vi "LV to ITX  Retrieve-HY.vi"(0 "File or Folder Path":path=path "P:/expt/PPMS 2 Data/SA03074H-20190112/08-IV curves-SG 2&3@0T", 5 "offset":i32, 7 "length":i32=91, 9 "index":T1={"A"=17, "B"=4, "C"=4, "D"=1, "E"=17, "N1"=3, "N2"=2, "N3"=0, "N4"=0}, 11 "stop":bool, 12 "file contains 2D data?":bool) -> (4 "A vs B":cluster{dbl[], dbl[]}[](graph), 6 "C vs D":cluster{dbl[], dbl[]}[](graph), 8 "E":dbl[][](graph), 10 "N":cluster{"N1":dbl, "N2":dbl, "N3":dbl, "N4":dbl}={"N1"=0.0, "N2"=0.0, "N3"=3631102351.878283, "N4"=3631102351.878283} {"N4" format="%#_6p"; "N3" format="%#_6p"; "N2" format="%#_6p"; "N1" format="%#_6p"}, 14 "Comments":string="IGOR\nX// Date: 1/23/2019 10:40 AM\nX// T sweep, B sweep, BG=11.5V\nX// \nX// T sweep: 4.5K, 5K, 5.5K\nX// B sweep: 7 to 0T, 0.2T step, 0.5T/min\nX// SG 3: 0 ac + dc: 365mV\nX// SG 2: 0 ac + dc: V(B)+(-450mV to 450mV), 0.5mV step, Ramp \nX// V(B)=V(0T)-17mV*|B|, V(0T)=300mV\nX// \nX// S-5:  2mV ac + 0 dc, 11Hz, Sinewave\nX// D-27\nX// V1+/-: 5/28\nX// \nX// prefilter: 60Hz prefilter-off\nX// TC: 500ms, order-2\nX// filter fC (Hz): 0.31831\nX// Vbg: 1\nX// \n\nX// Temp=5.500000\n\nX// \n\nX// B_Field=2.000000\n\nX// \n\nX// B_Field_Rate=0.500000\n\nX// \n\n\n\n\n\n\n\n\n\n\n\n\n\n\n\n\n\n\n\n\n\n\n\n\n\n\n\n\n\n\n\n\n\n\n\n\n\n\n\n\n\n\n\n\nX \nX Display/R 'time.SA03074H.000097'\nX AppendToGraph 'T.SA03074H.000097'\nX AppendToGraph 'B.SA03074H.000097'\nX AppendToGraph 'B_rate.SA03074H.000097'\nX AppendToGraph 'Vsg.SA03074H.000097'\nX AppendToGraph 'X0.SA03074H.000097'\nX AppendToGraph 'Y0.SA03074H.000097'\nX AppendToGraph 'X1.SA03074H.000097'\nX AppendToGraph 'Y1.SA03074H.000097'\nX AppendToGraph 'X2.SA03074H.000097'\nX AppendToGraph 'Y2.SA03074H.000097'\nX AppendToGraph 'X3.SA03074H.000097'\nX AppendToGraph 'Y3.SA03074H.000097'\nX AppendToGraph 'X4.SA03074H.000097'\nX AppendToGraph 'Y4.SA03074H.000097'\nX AppendToGraph 'X5.SA03074H.000097'\nX AppendToGraph 'Y5.SA03074H.000097'\nX AppendToGraph 'X6.SA03074H.000097'\nX AppendToGraph 'Y6.SA03074H.000097'\nX AppendToGraph 'X7.SA03074H.000097'\nX AppendToGraph 'Y7.SA03074H.000097'\nX Label bottom \"x label\"\nX Label left \"y label\"\nX ModifyGraph rgb('time.SA03074H.000097')=(65280,0,0)\nX ModifyGraph rgb('T.SA03074H.000097')=(65280,16896,0)\nX ModifyGraph rgb('B.SA03074H.000097')=(65280,33792,0)\nX ModifyGraph rgb('B_rate.SA03074H.000097')=(65280,50688,0)\nX ModifyGraph rgb('Vsg.SA03074H.000097')=(63488,65280,0)\nX ModifyGraph rgb('X0.SA03074H.000097')=(46592,65280,0)\nX ModifyGraph rgb('Y0.SA03074H.000097')=(29696,65280,0)\nX ModifyGraph rgb('X1.SA03074H.000097')=(12800,65280,0)\nX ModifyGraph rgb('Y1.SA03074H.000097')=(0,65280,4096)\nX ModifyGraph rgb('X2.SA03074H.000097')=(0,65280,20992)\nX ModifyGraph rgb('Y2.SA03074H.000097')=(0,65280,37888)\nX ModifyGraph rgb('X3.SA03074H.000097')=(0,65280,53248)\nX ModifyGraph rgb('Y3.SA03074H.000097')=(0,60928,65280)\nX ModifyGraph rgb('X4.SA03074H.000097')=(0,44032,65280)\nX ModifyGraph rgb('Y4.SA03074H.000097')=(0,27136,65280)\nX ModifyGraph rgb('X5.SA03074H.000097')=(0,10240,65280)\nX ModifyGraph rgb('Y5.SA03074H.000097')=(6656,0,65280)\nX ModifyGraph rgb('X6.SA03074H.000097')=(23552,0,65280)\nX ModifyGraph rgb('Y6.SA03074H.000097')=(40448,0,65280)\nX ModifyGraph rgb('X7.SA03074H.000097')=(57344,0,65280)\nX ModifyGraph rgb('Y7.SA03074H.000097')=(65280,0,56832)\nX Legend/C/N=text0/J \"\\\\s('time.SA03074H.000097') time\\r\\\\s('T.SA03074H.000097') T\\r\\\\s('B.SA03074H.000097') B\\r\\\\s('B_rate.SA03074H.000097') B_rate\\r\\\\s('Vsg.SA03074H.000097') Vsg\\r\\\\s('X0.SA03074H.000097') X0\\r\\\\s('Y0.SA03074H.000097') Y0\\r\\\\s('X1.SA03074H.000097') X1\\r\\\\s('Y1.SA03074H.000097') Y1\\r\\\\s('X2.SA03074H.000097') X2\\r\\\\s('Y2.SA03074H.000097') Y2\\r\\\\s('X3.SA03074H.000097') X3\\r\\\\s('Y3.SA03074H.000097') Y3\\r\\\\s('X4.SA03074H.000097') X4\\r\\\\s('Y4.SA03074H.000097') Y4\\r\\\\s('X5.SA03074H.000097') X5\\r\\\\s('Y5.SA03074H.000097') Y5\\r\\\\s('X6.SA03074H.000097') X6\\r\\\\s('Y6.SA03074H.000097') Y6\\r\\\\s('X7.SA03074H.000097') X7\\r\\\\s('Y7.SA03074H.000097') Y7\"\nX ModifyGraph mirror(bottom)=1\nX ModifyGraph width=216\nX ModifyGraph height={Aspect,0.6}\nX ModifyGraph Log(bottom)=0\nX ModifyGraph Log(left)=0\nX \n")   [LabVIEW 2016]
uses:
  <vilib>/Utility/miscctls.llb/LVOffsetAndMultiplierTypeDef.ctl
  <userlib>/LevyLab/LV to ITX/LVtoITX.lvclass
  <vilib>/Analysis/NI_AALPro.lvlib
panel:
  in  "Offset value":dbl
  in  "Add offset?":bool
  out "size(s)":i32[](array[numeric])=[21, 1801]
  in  "Specify data section ?":bool
  in  "Data length":i32=5000
  in  "Data offset":i32
  in  "Tab Control 2":enum32{"Amplifier settings", "Page 2"}(tab)
  in  "Sensitivity":dbl
  in  "Current gain":dbl
  out "Actual Current Multiplier (A)":dbl=nan
  in  "Voltage gain":dbl
  in  "Exciting voltage":dbl
  out "Actual Conductance Multiplier (S)":dbl=nan
  out "Actual Conductance Multiplier (e2/h)":dbl=nan
  in  "Unit of conductance":u16(ring) items=["Unit: e2/h", "Unit: S", "Multiplier: 1", "Multiplier: Manual input"]
  in  "Manual input":dbl
  in  "Tab Control":enum32{"Curve-Vertical", "Curve-Horizontal"}(tab)=enum."Curve-Horizontal"
  out "Drag V":cluster{dbl[], dbl[]}(graph)={[7.0, 6.8, 6.6, 6.4, 6.2, 6.0, 5.8, 5.6, 5.4, 5.2, 5.0, 4.8, 4.6, 4.4, 4.199999999999999, 4.0, 3.8, 3.5999999999999996, 3.4, 3.1999999999999997, 3.0, 2.8, 2.5999999999999996, 2.3999999999999995, 2.1999999999999993, 2.0], [nan, nan, nan, nan, nan, nan, nan, nan, nan, nan, nan, nan, nan, nan, nan, nan, nan, nan, nan, nan, nan, nan, nan, nan, nan, nan]}
  out "Numeric X":i32=1
  in  "Average width X":i32=1
  out "From X":dbl=-0.2832407407407408 format="%#_4p"
  out "To X":dbl=-0.2827407407407408 format="%#_4p"
  out "Drag V 2":cluster{dbl[], dbl[]}(graph)={[-0.45, -0.4495, -0.449, -0.4485, -0.448, -0.4475, -0.447, -0.4465, -0.446, -0.4455, -0.445, -0.4445, -0.444, -0.4435, -0.443, -0.4425, -0.442, -0.4415, -0.441, -0.4405, -0.44, -0.4395, -0.439, -0.4385, -0.438, -0.4375], [nan, nan, nan, nan, nan, nan, nan, nan, nan, nan, nan, nan, nan, nan, nan, nan, nan, nan, nan, nan, nan, nan, nan, nan, nan, nan]}
  out "Numeric Y":i32=21
  out "To Y":dbl=-0.3885714285714288 format="%#_4p"
  out "From  Y":dbl=3.8114285714285714 format="%#_4p"
  in  "Average width Y":i32=21
  out "Y Scale Multiplier":dbl=1.0
  out "Z Scale Multiplier":dbl=1.0
  in  "D  is time?":bool
  in  "B is time?":bool
  out "time":string[][](table)=[["1/23/2019", "6:37 AM"], ["1/23/2019", "6:47 AM"], ["1/23/2019", "6:57 AM"], ["1/23/2019", "7:07 AM"], ["1/23/2019", "7:16 AM"], ["1/23/2019", "7:26 AM"], ["1/23/2019", "7:36 AM"], ["1/23/2019", "7:45 AM"], ["1/23/2019", "7:55 AM"], ["1/23/2019", "8:05 AM"], ["1/23/2019", "8:15 AM"], ["1/23/2019", "8:24 AM"], ["1/23/2019", "8:34 AM"], ["1/23/2019", "8:44 AM"], ["1/23/2019", "8:54 AM"], ["1/23/2019", "9:03 AM"], ["1/23/2019", "9:13 AM"], ["1/23/2019", "9:23 AM"], ["1/23/2019", "9:32 AM"], ["1/23/2019", "9:42 AM"], ["1/23/2019", "9:52 AM"], ["1/23/2019", "10:02 AM"], ["1/23/2019", "10:11 AM"], ["1/23/2019", "10:21 AM"], ["1/23/2019", "10:31 AM"], ["1/23/2019", "10:40 AM"]]
  in  "Use Folder Index File?":bool
  in  "Generate Folder Index File?":bool
  in  "Ez name":string="I (A)"
  in  "Ey name":string="B (T)"
  in  "Ex name":string="(DC of SG-L)-V(B) (V)"
  in  "C y name":string="C y name"
  in  "D x name":string="D x name"
  in  "A y name":string="I (A)"
  in  "B x name":string="(DC of SG-L)-V(B) (V)"
  out "Index, Wavenames":string[][](table)=[["0", "'time.SA03074H.000097'\n"], ["1", "'T.SA03074H.000097'\n"], ["2", "'B.SA03074H.000097'\n"], ["3", "'B_rate.SA03074H.000097'\n"], ["4", "'Vsg.SA03074H.000097'\n"], ["5", "'X0.SA03074H.000097'\n"], ["6", "'Y0.SA03074H.000097'\n"], ["7", "'X1.SA03074H.000097'\n"], ["8", "'Y1.SA03074H.000097'\n"], ["9", "'X2.SA03074H.000097'\n"], ["10", "'Y2.SA03074H.000097'\n"], ["11", "'X3.SA03074H.000097'\n"], ["12", "'Y3.SA03074H.000097'\n"], ["13", "'X4.SA03074H.000097'\n"], ["14", "'Y4.SA03074H.000097'\n"], ["15", "'X5.SA03074H.000097'\n"], ["16", "'Y5.SA03074H.000097'\n"], ["17", "'X6.SA03074H.000097'\n"], ["18", "'Y6.SA03074H.000097'\n"], ["19", "'X7.SA03074H.000097'\n"], ["20", "'Y7.SA03074H.000097'\n"], ["", ""]]
  in  "recolor traces?":bool
  in  "Ex":T2={"Offset"=-0.45, "Multiplier"=0.0005}
  in  "Ey":T2={"Offset"=7.0, "Multiplier"=-0.2}
  out "Path":path=path "P:/expt/PPMS 2 Data/SA03074H-20190112/11A-SG-L sweep at B 4K~6K/SA03074H.000097.itx"
  out "counter":i32=25
  in  "pattern":string="*.itx"
  # "Add offset to curves?"
  # "Specify data section"
  # "Setting for Conductance caculation"
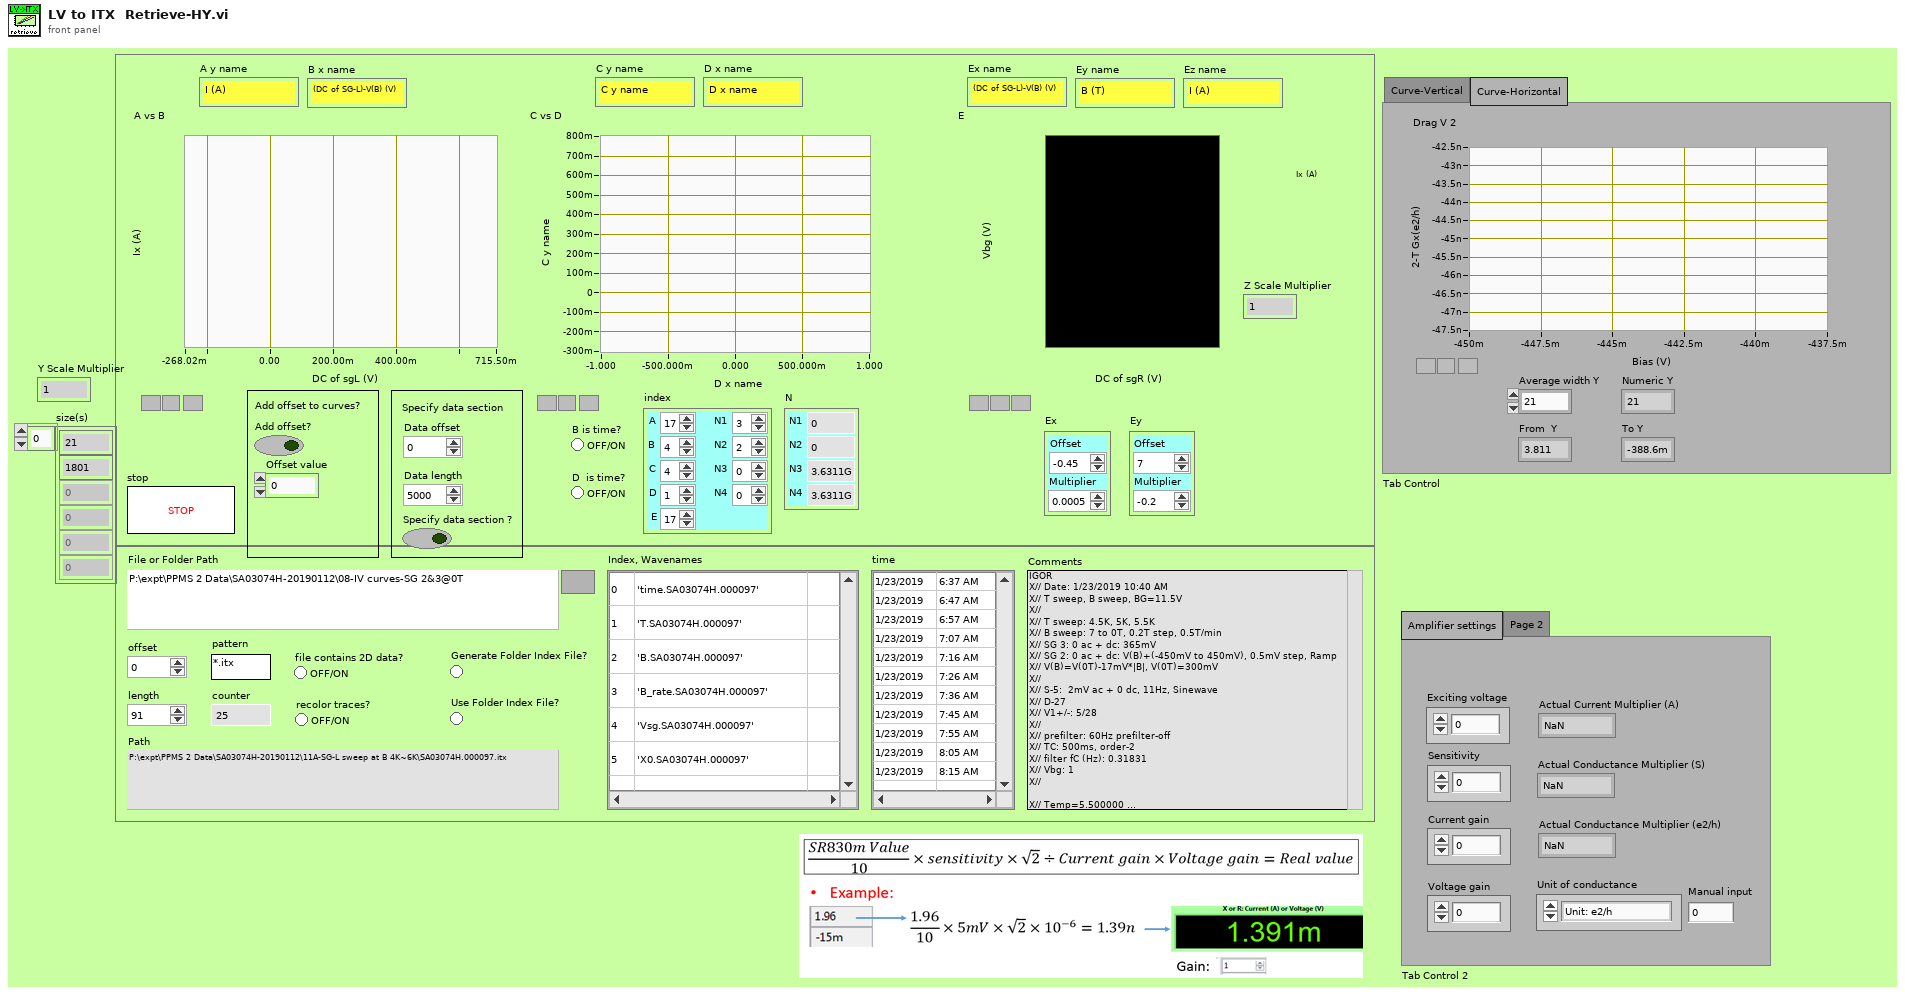
[diagram p1: front panel]
types:
  T1 = cluster{"A":i32, "B":i32, "C":i32, "D":i32, "E":i32, "N1":i32, "N2":i32, "N3":i32, "N4":i32}
  T2 = typedef "LVOffsetAndMultiplierTypeDef.ctl" = cluster{"Offset":dbl, "Multiplier":dbl}
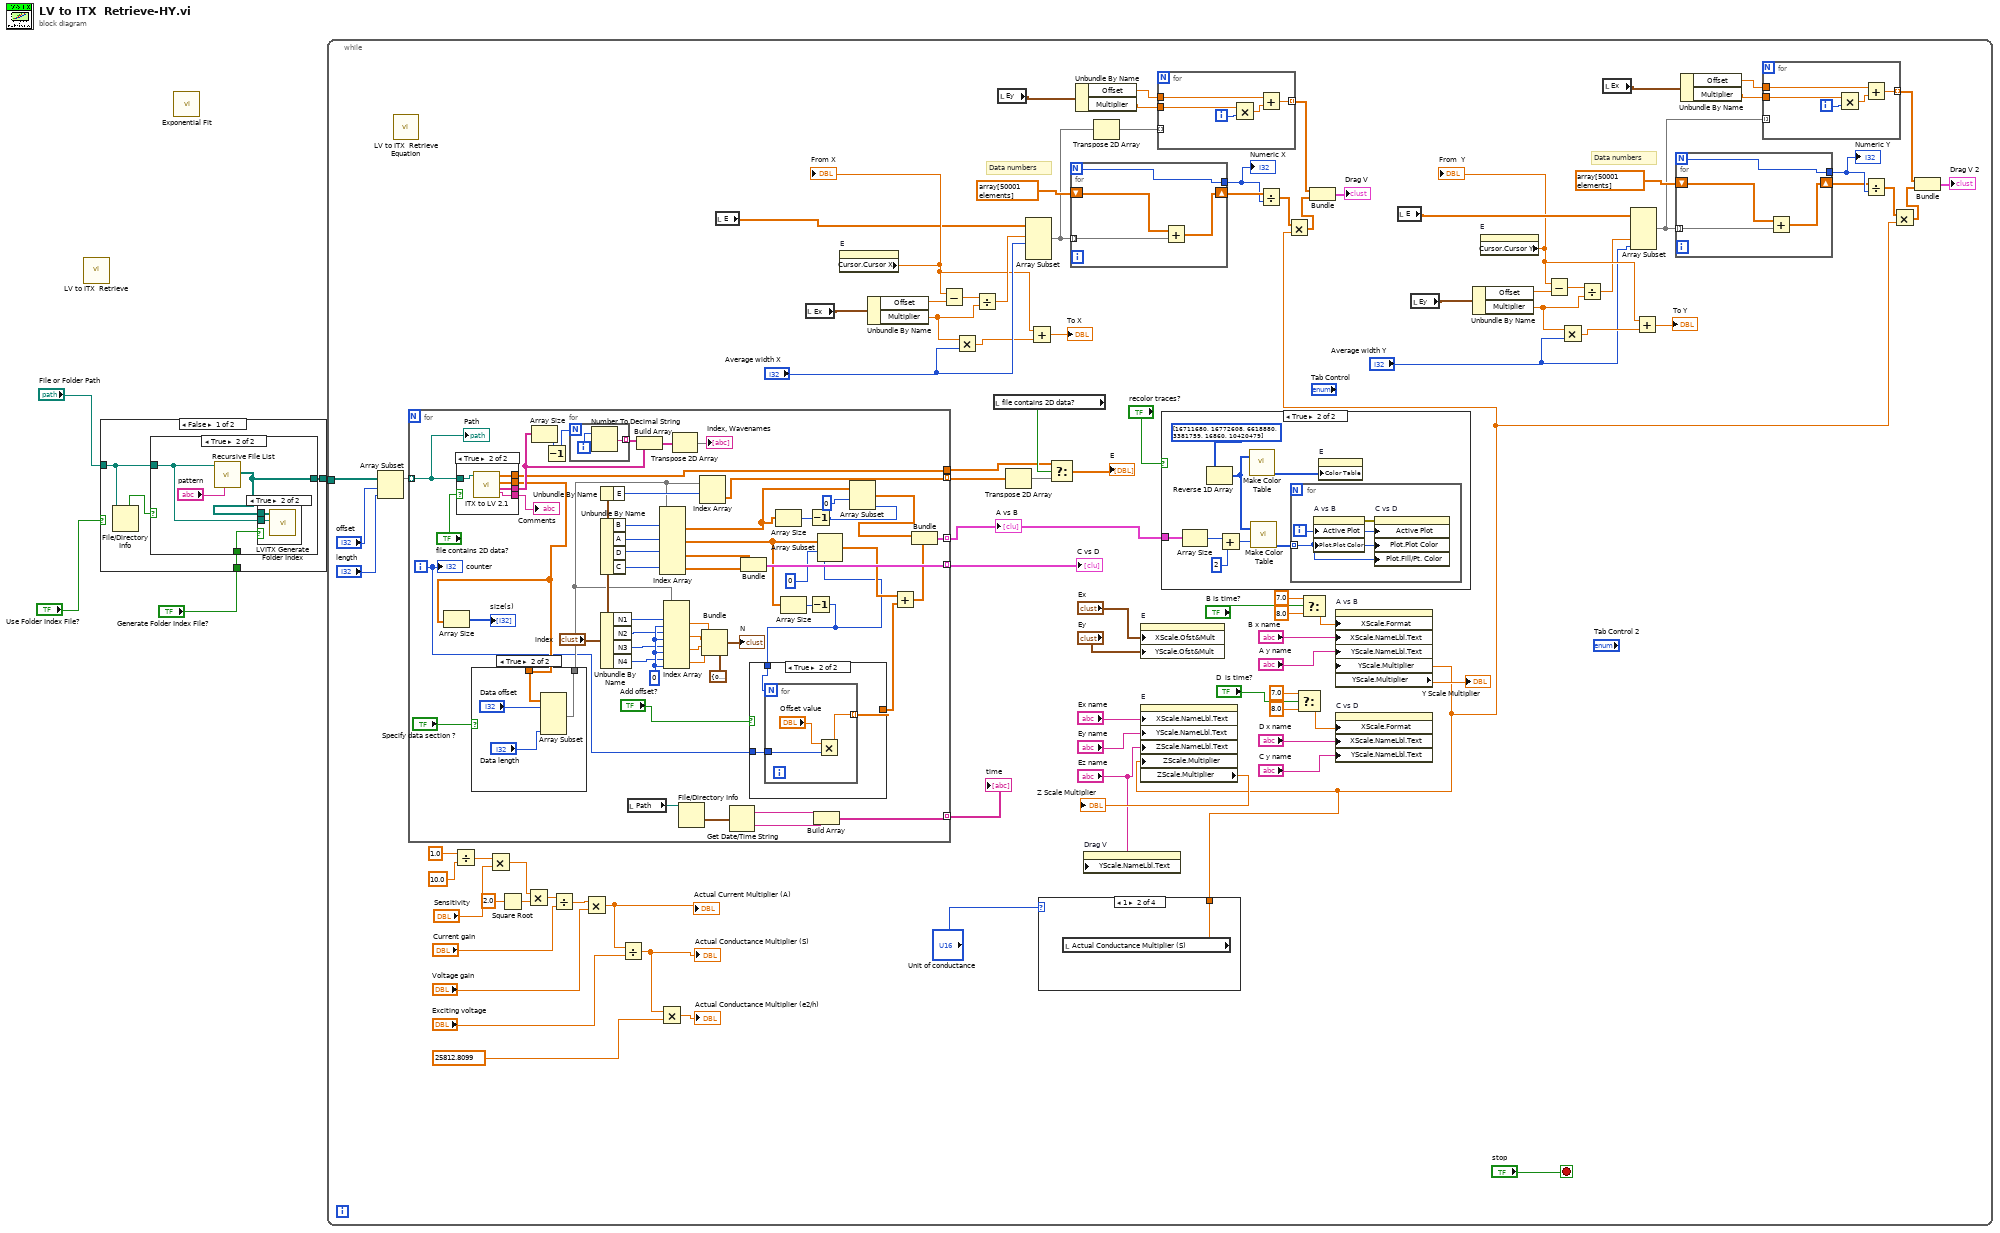
[diagram p0: block diagram]
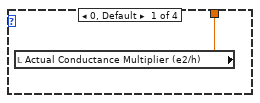
[diagram p2: hidden frame]
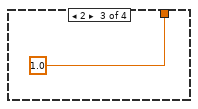
[diagram p3: hidden frame]
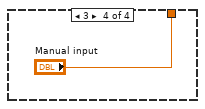
[diagram p4: hidden frame]
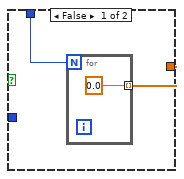
[diagram p6: hidden frame]
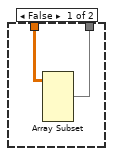
[diagram p7: hidden frame]
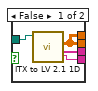
[diagram p8: hidden frame]
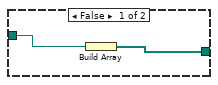
[diagram p9: hidden frame]
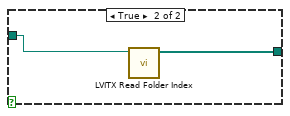
[diagram p11: hidden frame]
diagram:
  n1 = call <userlib>:"LV to ITX  Retrieve.vi"() -> ()  [unwired: 11 in, 5 out]
  n2 = case shown="False" "Use Folder Index File?" {
    tunnel: [w6 w17] -> w2
    tunnel: "File or Folder Path" -> [w8 w18]
    tunnel: "Generate Folder Index File?" -> [w5 _]
    frame False {
      n3 = File/Directory Info(path=w8) -> (directory=w7:bool)  [unwired: 1 in, 6 out]
      n4 = case shown="True" w7 {
        tunnel: [w10 w13] -> w6
        tunnel: w8 -> [w9 w12]
        tunnel: w5 -> [_ w11]
        frame False {
          n5 = Build Array(w9) -> (w10:path[])
        }
        frame True {
          n6 = call <vilib>:"Recursive File List.vi"("pattern"="pattern", "Folder Path"=w12) -> ("All Files in Dir"=w13:path[])  [unwired: 5 in, 4 out]
          n7 = case shown="True" w11 {
            tunnel: w13 -> [_ w16]
            tunnel: w12 -> [_ w15]
            frame False {
            }
            frame True {
              n8 = call <userlib>:"LVITX Generate Folder Index.vi"("File or Folder Path"=w15, "All Files in Dir"=w16) -> ()  [unwired: 9 in, 1 out]
            }
          }
        }
      }
    }
    frame True {
      n9 = call <userlib>:"LVITX Read Folder Index.vi"("File or Folder Path"=w18) -> ("Files"=w17:path[])  [unwired: 9 in, 1 out]
    }
  }
  n10 = call <vilib>:"Exponential Fit.vi"() -> ()  [unwired: 10 in, 6 out]
  n11 = while {
    tunnel: w2 -> [w95]
    stop <- "stop" stop-if-true
    # "Data numbers"
    # "Data numbers"
    n12 = Array Subset(array=w95, index="offset", length="length") -> (w94:path[])
    n13 = call <userlib>:"LV to ITX  Retrieve Equation.vi"() -> ()  [unwired: 11 in, 5 out]
    n14 = for {
      tunnel: w94 -> [w199] mode=indexing
      tunnel: [w199] -> _ mode=indexing
      tunnel: [w198] -> w22 mode=indexing
      tunnel: [w196] -> w105 mode=indexing
      tunnel: [w173] -> w109 mode=indexing
      tunnel: [w187] -> w107
      tunnel: [w164] -> w98 mode=indexing
      i -> [w149]
      w186 = 0 ("disabled index (col)")
      n15 = case shown="True" "file contains 2D data?" {
        tunnel: [w221 w224] -> w200
        tunnel: [w219 w225] -> w152
        tunnel: w199 -> [w220 w226]
        tunnel: [w218 w223] -> w188
        tunnel: [w219 w222] -> w187
        frame False {
          n16 = call <userlib>:"ITX to LV 2.1 1D.vi"("file (use dialog)"=w220) -> ("wave names"=w218:string[], "1D arrays"=w219:dbl[][], "Notes"=w221:string)  [unwired: 6 in, 2 out]
        }
        frame True {
          n17 = call <userlib>:"ITX to LV 2.1.vi"("file (use dialog)"=w226) -> ("wave names"=w223:string[], "1D arrays"=w225:dbl[][], "2D array"=w222:dbl[][], "Notes"=w224:string)  [unwired: 6 in, 1 out]
        }
      }
      "Comments" <- w200
      n18 = Array Size(array=w152) -> (size(s)=→"size(s)":i32[])
      n19 = case shown="True" "Specify data section ?" {
        tunnel: w152 -> [w211 w215]
        tunnel: [w210 w214] -> w155
        frame False {
          n20 = Array Subset(array=w211) -> (w210:dbl[][])  [unwired: 4 in]
        }
        frame True {
          n21 = Array Subset(array=w215, index (col)="Data offset", length (col)="Data length") -> (w214:dbl[][])  [unwired: 2 in]
        }
      }
      n22 = Array Size(array=w188) -> (size(s)=w191:i32)
      n23 = Decrement(x=w191) -> (x-1=w190:i32)
      n24 = for {
        N: w190 -> [_]
        tunnel: [w216] -> w194 mode=indexing
        i -> [w217]
        n25 = Number To Decimal String(number=w217) -> (decimal integer string=w216:string)  [unwired: 1 in]
      }
      n26 = Unbundle By Name("index") -> ("E"=w178:i32)
      n27 = Unbundle By Name("index") -> ("B"=w177:i32, "A"=w176:i32, "D"=w175:i32, "C"=w174:i32)
      n28 = Unbundle By Name("index") -> ("N1"=w179:i32, "N2"=w180:i32, "N3"=w181:i32, "N4"=w182:i32)
      n29 = local read "Path"() -> (w171:path)
      n30 = Build Array(w194, w188) -> (w189:string[][])
      n31 = Index Array(array=w155, index (row) #1=w177, index (row) #2=w176, index (row) #3=w175, index (row) #4=w174) -> (element #1=w163:dbl[], element #2=w157:dbl[], element #3=w192:dbl[], element #4=w195:dbl[])  [unwired: 4 in]
      n32 = Index Array(array=w155, index (row) #1=w179, index (col) #1=w186, index (row) #2=w180, index (col) #2=w186, index (row) #3=w181, index (col) #3=w186, index (row) #4=w182, index (col) #4=w186) -> (element #1=w168:dbl, element #2=w169:dbl, element #3=w170:dbl, element #4=w185:dbl)
      n33 = Transpose 2D Array(2D array=w189) -> (transposed array=→"Index, Wavenames":string[][])
      n34 = File/Directory Info(path=w171) -> (last mod=w167:timestamp)  [unwired: 1 in, 6 out]
      n35 = Index Array(array=w155, index (row)=w178) -> (element=w173:dbl[])  [unwired: 1 in]
      n36 = Bundle(cluster=cluster{"N1":dbl, "N2":dbl, "N3":dbl, "N4":dbl} {"N1"=0.0, "N2"=0.0, "N3"=0.0, "N4"=0.0}, "N1"=w168, "N2"=w169, "N3"=w170, "N4"=w185) -> (→"N":cluster{"N1":dbl, "N2":dbl, "N3":dbl, "N4":dbl})
      n37 = Get Date/Time String(seconds (now)=w167) -> (date string=w166:string, time string=w165:string)  [unwired: 2 in]
      n38 = Bundle(w192, w195) -> (w196:cluster{dbl[], dbl[]})  [unwired: 1 in]
      n39 = Array Size(array=w163) -> (size(s)=w162:i32)
      n40 = Array Size(array=w157) -> (size(s)=w159:i32)
      n41 = Decrement(x=w162) -> (x-1=w156:i32)
      n42 = Decrement(x=w159) -> (x-1=w148:i32)
      n43 = case shown="True" "Add offset?" {
        tunnel: [w202 w206] -> w146
        tunnel: w149 -> [_ w205]
        tunnel: w148 -> [w201 w204]
        frame False {
          n44 = for {
            N: w201 -> [_]
            tunnel: [0.0] -> w202 mode=indexing
          }
        }
        frame True {
          n45 = for {
            N: w204 -> [_]
            tunnel: [w209] -> w206 mode=indexing
            tunnel: w205 -> [w207]
            n46 = Multiply(x="Offset value", y=w207) -> (x*y=w209:dbl)
          }
        }
      }
      n47 = Build Array(w166, w165) -> (w164:string[])
      n48 = Array Subset(array=w157, index=0, length=w148) -> (w151:dbl[])
      n49 = Array Subset(array=w163, index=0, length=w156) -> (w160:dbl[])
      n50 = Add(x=w151, y=w146) -> (x+y=w150:dbl[])
      n51 = Bundle(w160, w150) -> (w198:cluster{dbl[], dbl[]})  [unwired: 1 in]
      "counter" <- w149
      "Path" <- w199
    }
    "A vs B" <- w22
    "C vs D" <- w105
    "time" <- w98
    n52 = Divide(x=1.0 ("y"), y=10.0) -> (x/y=w80:dbl)
    n53 = Multiply(x=w80, y="Sensitivity") -> (x*y=w79:dbl)
    n54 = Square Root(x=2.0) -> (sqrt(x)=w78:dbl)
    n55 = Multiply(x=w79, y=w78) -> (x*y=w77:dbl)
    n56 = Divide(x=w77, y="Current gain") -> (x/y=w76:dbl)
    n57 = Multiply(x=w76, y="Voltage gain") -> (x*y=w74:dbl)
    "Actual Current Multiplier (A)" <- w74
    n58 = Divide(x=w74, y="Exciting voltage") -> (x/y=w68:dbl)
    "Actual Conductance Multiplier (S)" <- w68
    n59 = Multiply(x=w68, y=25812.8099) -> (x*y=→"Actual Conductance Multiplier (e2/h)":dbl)
    n60 = local read "E"() -> (w42:dbl[][])
    n61 = local read "Ex"() -> (w43:T2)
    n62 = property on="E" class="IntGraph (strict)"() -> ("Cursor.Cursor X"=w48:dbl)  [unwired: 2 in, 2 out]
    "From X" <- w48
    n63 = Unbundle By Name(w43) -> ("Offset"=w59:dbl, "Multiplier"=w51:dbl)
    n64 = Subtract(x=w48, y=w59) -> (x-y=w65:dbl)
    n65 = Multiply(x=w51, y="Average width X") -> (x*y=w49:dbl)
    n66 = Divide(x=w65, y=w51) -> (x/y=w64:dbl)
    n67 = local read "file contains 2D data?"() -> (w111:bool)
    n68 = local read "Ey"() -> (w44:T2)
    n69 = Transpose 2D Array(2D array=w109) -> (transposed array=w110:dbl[][])
    n70 = Array Subset(array=w42, index (row)=w64, length (row)="Average width X") -> (w61:dbl[][])  [unwired: 2 in]
    n71 = Add(x=w48, y=w49) -> (x+y=→"To X":dbl)
    n72 = case shown="1" "Unit of conductance" {
      tunnel: [w131 w132 1.0 "Manual input"] -> w23
      frame 0, Default {
        n73 = local read "Actual Conductance Multiplier (e2/h)"() -> (w131:dbl)
      }
      frame 1 {
        n74 = local read "Actual Conductance Multiplier (S)"() -> (w132:dbl)
      }
      frame 2 {
      }
      frame 3 {
      }
    }
    n75 = Select(t=w107, s=w111, f=w110) -> (s? t:f=→"E":dbl[][])
    n76 = for {
      N -> [w127]
      tunnel: w61 -> [w130] mode=indexing
      shift-right: [w129] -> w62
      shift-left: dbl[] array[50001 elements] -> [w128]
      tunnel: [w127] -> w45
      n77 = Add(x=w128, y=w130) -> (x+y=w129:dbl[])
    }
    "Numeric X" <- w45
    n78 = Unbundle By Name(w44) -> ("Offset"=w56:dbl, "Multiplier"=w55:dbl)
    n79 = property on="Drag V" class="XYGraph (strict)"("YScale.NameLbl.Text"="Ez name") -> ()  [unwired: 2 in, 2 out]
    n80 = Transpose 2D Array(2D array=w61) -> (transposed array=w60:dbl[][])
    n81 = property on="E" class="IntGraph (strict)"("XScale.Ofst&Mult"="Ex", "YScale.Ofst&Mult"="Ey") -> ()  [unwired: 2 in, 2 out]
    n82 = property on="E" class="IntGraph (strict)"("XScale.NameLbl.Text"="Ex name", "YScale.NameLbl.Text"="Ey name", "ZScale.NameLbl.Text"="Ez name", "ZScale.Multiplier"=w23) -> ("ZScale.Multiplier"=→"Z Scale Multiplier":dbl)  [unwired: 2 in, 2 out]
    n83 = for {
      tunnel: w60 -> [_] mode=indexing
      tunnel: w56 -> [w125]
      tunnel: [w123] -> w58 mode=indexing
      tunnel: w55 -> [w122]
      i -> [w126]
      n84 = Multiply(x=w122, y=w126) -> (x*y=w124:dbl)
      n85 = Add(x=w125, y=w124) -> (x+y=w123:dbl)
    }
    n86 = case shown="True" "recolor traces?" {
      tunnel: w22 -> [_ w137]
      frame False {
      }
      frame True {
        n87 = Array Size(array=w137) -> (size(s)=w138:i32)
        n88 = Reverse 1D Array(array=u32[] [16711680, 16772608, 6618880, 3381759, 16860, 10420479] ("color scale")) -> (reversed array=w136:u32[])
        n89 = Add(x=w138, y=2 ("x")) -> (x+y=w142:i32)
        n90 = call <userlib>:"Make Color Table.vi"("Array"=w136) -> ("Color Tbl"=w140:u32[])  [unwired: 1 in, 3 out]
        n91 = call <userlib>:"Make Color Table.vi"("Array"=w136, "Size"=w142) -> ("Color Tbl"=w139:u32[])  [unwired: 3 out]
        n92 = for {
          tunnel: w139 -> [w143] mode=indexing
          i -> [w144]
          n93 = property on="A vs B" class="XYGraph (strict)"("Active Plot"=w144, "Plot.Plot Color"=w143) -> (error out=w145:errorcluster)  [unwired: 2 in, 1 out]
          n94 = property on="C vs D" class="XYGraph (strict)"(error in=w145, "Active Plot"=w144, "Plot.Plot Color"=w143, "Plot.Fill/Pt. Color"=w143) -> ()  [unwired: 1 in, 2 out]
        }
        n95 = property on="E" class="IntGraph (strict)"("Color Table"=w140) -> ()  [unwired: 2 in, 2 out]
      }
    }
    n96 = Divide(x=w62, y=w45) -> (x/y=w53:dbl[])
    n97 = Multiply(x=w53, y=w23) -> (x*y=w52:dbl[])
    n98 = Select(t=7.0, s="D  is time?", f=8.0) -> (s? t:f=w90:dbl)
    n99 = Select(t=7.0, s="B is time?", f=8.0) -> (s? t:f=w91:dbl)
    n100 = Bundle(w58, w52) -> (→"Drag V":cluster{dbl[], dbl[]})  [unwired: 1 in]
    n101 = property on="A vs B" class="XYGraph (strict)"("XScale.Format"=w91, "XScale.NameLbl.Text"="B x name", "YScale.NameLbl.Text"="A y name", "YScale.Multiplier"=w23) -> ("YScale.Multiplier"=→"Y Scale Multiplier":dbl)  [unwired: 2 in, 2 out]
    n102 = property on="C vs D" class="XYGraph (strict)"("XScale.Format"=w90, "XScale.NameLbl.Text"="D x name", "YScale.NameLbl.Text"="C y name") -> ()  [unwired: 2 in, 2 out]
    n103 = local read "E"() -> (w41:dbl[][])
    n104 = local read "Ey"() -> (w40:T2)
    n105 = Unbundle By Name(w40) -> ("Offset"=w27:dbl, "Multiplier"=w34:dbl)
    n106 = property on="E" class="IntGraph (strict)"() -> ("Cursor.Cursor Y"=w36:dbl)  [unwired: 2 in, 2 out]
    "From  Y" <- w36
    n107 = Subtract(x=w36, y=w27) -> (x-y=w24:dbl)
    n108 = Multiply(x=w34, y="Average width Y") -> (x*y=w35:dbl)
    n109 = Divide(x=w24, y=w34) -> (x/y=w20:dbl)
    n110 = local read "Ex"() -> (w39:T2)
    n111 = Array Subset(array=w41, index (col)=w20, length (col)="Average width Y") -> (w19:dbl[][])  [unwired: 2 in]
    n112 = Add(x=w36, y=w35) -> (x+y=→"To Y":dbl)
    n113 = for {
      N -> [w118]
      tunnel: w19 -> [w121] mode=indexing
      shift-right: [w120] -> w26
      shift-left: dbl[] array[50001 elements] -> [w119]
      tunnel: [w118] -> w38
      n114 = Add(x=w119, y=w121) -> (x+y=w120:dbl[])
    }
    "Numeric Y" <- w38
    n115 = Unbundle By Name(w39) -> ("Offset"=w30:dbl, "Multiplier"=w31:dbl)
    n116 = for {
      tunnel: w19 -> [_] mode=indexing
      tunnel: w30 -> [w116]
      tunnel: [w114] -> w28 mode=indexing
      tunnel: w31 -> [w113]
      i -> [w117]
      n117 = Multiply(x=w113, y=w117) -> (x*y=w115:dbl)
      n118 = Add(x=w116, y=w115) -> (x+y=w114:dbl)
    }
    n119 = Divide(x=w26, y=w38) -> (x/y=w32:dbl[])
    n120 = Multiply(x=w32, y=w23) -> (x*y=w33:dbl[])
    n121 = Bundle(w28, w33) -> (→"Drag V 2":cluster{dbl[], dbl[]})  [unwired: 1 in]
  }
